vi "Fetch from Buffer (Single Point).vi"(8 "error in (no error)":errorcluster, 9 "Buffer Elements":u16(ring) items=["Date", "Extra", "Formatted", "Fractional", "Relative", "Seconds", "Status", "Time", "Timestamp", "Unit"], 10 "Buffer Name":string="defbuffer1", 11 "VISA resource name":refnum<visa-resource-name>) -> (0 "error out":errorcluster, 1 "Element Value":string, 2 "Measurement":dbl, 3 "VISA resource name out":refnum<visa-resource-name>)   [LabVIEW 2015, in "Keithley DMM7510.lvlib"]
doc: "Reads and returns a single measurement from the instrument."
uses:
  Keithley DMM7510.lvlib
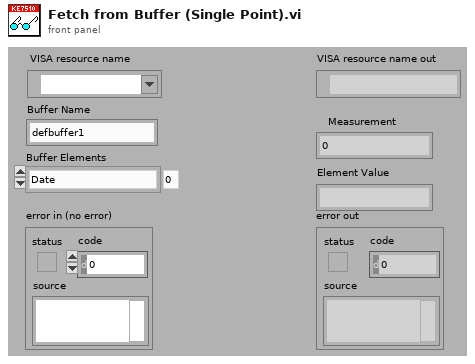
[diagram p1: front panel]
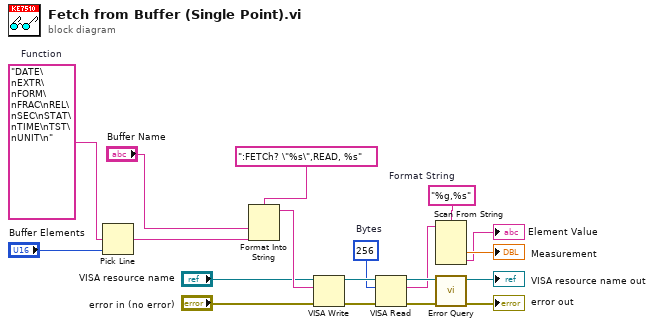
[diagram p0: block diagram]
diagram:
  w5 = "DATE\nEXTR\nFORM\nFRAC\nREL\nSEC\nSTAT\nTIME\nTST\nUNIT\n"  # Function
  w11 = "%g,%s"  # Format String
  w17 = u32 256  # Bytes
  n1 = Pick Line(multi-line string=w5, line index="Buffer Elements") -> (output string=w4:string)  [unwired: 1 out]
  n2 = Format Into String(format string=":FETCh? \"%s\",READ, %s", "Buffer Name", w4) -> (resulting string=w10:string)  [unwired: 2 in, 1 out]
  n3 = VISA Write(VISA resource name="VISA resource name", write buffer=w10, error in (no error)="error in (no error)") -> (VISA resource name out=w18:refnum<visa-resource-name>, error out=w19:errorcluster)  [unwired: 1 out]
  n4 = VISA Read(VISA resource name=w18, byte count=w17, error in (no error)=w19) -> (VISA resource name out=w16:refnum<visa-resource-name>, read buffer=w12:string, error out=w15:errorcluster)  [unwired: 1 out]
  n5 = Scan From String(format string=w11, input string=w12) -> (output 1=→"Measurement":dbl, output 2=→"Element Value":string)  [unwired: 4 in, 3 out]
  n6 = call "Error Query.vi"("error in (no error)"=w15, "VISA resource name"=w16) -> ("error out"=→"error out":errorcluster, "VISA resource name out"=→"VISA resource name out":refnum<visa-resource-name>)  [unwired: 6 in, 2 out]
